vi "GetParam.vi"(8 "error in (no error)":errorcluster caption="entrée d'erreur (pas d'erreur)", 11 "Pairwise_distances_chunked.lvclass":refnum<class "Pairwise_distances_chunked.lvclass">) -> (0 "error out":errorcluster caption="sortie d'erreur", 2 "pairwise_distances_chunked":T1={"reduce_func"="None", "metric "="euclidean", "n_jobs"="None", "working_memory"="None"}, 3 "Pairwise_distances_chunked.lvclass":refnum<class "Pairwise_distances_chunked.lvclass">)   [LabVIEW 2020, in "Pairwise_distances_chunked.lvclass"]
doc: "Get Parameters"
uses:
  Pairwise_distances_chunked.lvclass
  Pairwise_distances_chunked.lvclass/Pairwise_distances_chunked.ctl
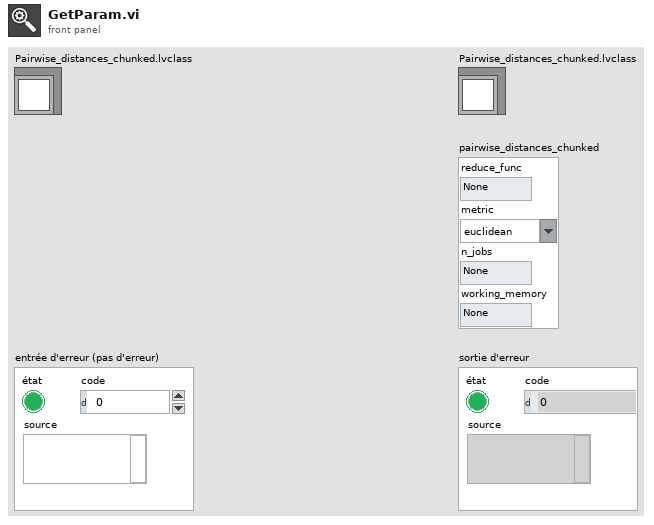
[diagram p1: front panel]
types:
  T1 = cluster{"reduce_func":string, "metric ":string, "n_jobs":string, "working_memory":string}
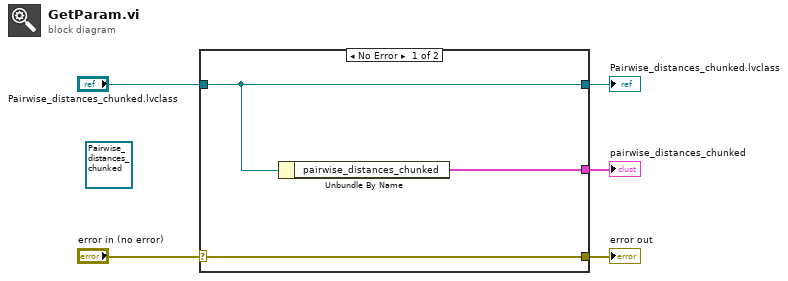
[diagram p0: block diagram]
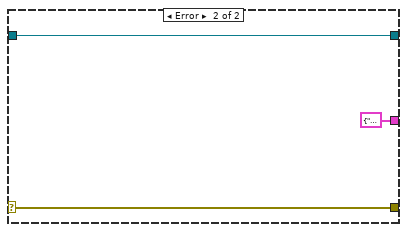
[diagram p2: hidden frame]
diagram:
  (unwired) refnum<class "Pairwise_distances_chunked.lvclass"> refnum ("Pairwise_distances_chunked.lvclass")
  n1 = case shown="No Error" "error in (no error)" {
    selector: "error in (no error)" -> [w8 w10]
    tunnel: [w8 w10] -> w4
    tunnel: [w7 w11] -> w2
    tunnel: "Pairwise_distances_chunked.lvclass" -> [w7 w11]
    tunnel: [w6 T1 {"reduce_func"="", "metric "="", "n_jobs"="", "working_memory"=""} ("pairwise_distances_chunked")] -> w1
    frame No Error {
      n2 = Unbundle By Name(w7) -> ("pairwise_distances_chunked"=w6:T1)
    }
    frame Error {
    }
  }
  "error out" <- w4
  "Pairwise_distances_chunked.lvclass" <- w2
  "pairwise_distances_chunked" <- w1
